vi "Device.Init.vi"(8 "error in (no error)":errorcluster, 11 "LIA.SR810":refnum<class "LIA.SR810.lvclass">) -> (0 "error out":errorcluster, 2 "Result":bool, 3 "LIA.SR810 out":refnum<class "LIA.SR810.lvclass">)   [LabVIEW 2017, in "LIA.SR810.lvclass"]
doc: "---------------------------------------------------------------\nJKI State Machine Objects™\nhttp://jki.net/state-machine-objects/\nCopyright (C) 2005-2015, JKI <info@jki.net>\nALL RIGHTS RESERVEDJKI State Machine Objects (SMO) 1.0.0.5\nJKI - JKI\nCopyright (c) 2016, JKI"
uses:
  LIA.SR810.lvclass
  D:/upwork/Laser Measurement Tool/Laser/project/Subsystems/LIA/LIA.lvclass
  Typedefs/Resource--Cluster.ctl
  LIA/LIA.lvclass
  <instrlib>/Stanford Research 830/Stanford Research 830.lvlib
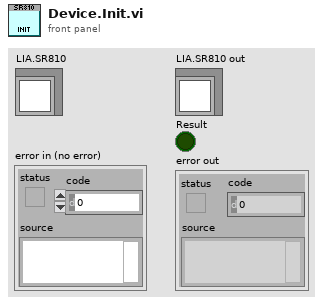
[diagram p1: front panel]
types:
  T1 = typedef "LIA.SR810.lvclass/Resource--Cluster.ctl" = cluster{"VISA resource":refnum<visa-resource-name>}
  T2 = typedef "LIA.lvclass/Configuration--Cluster.ctl" = cluster{"VISA Resource":string}
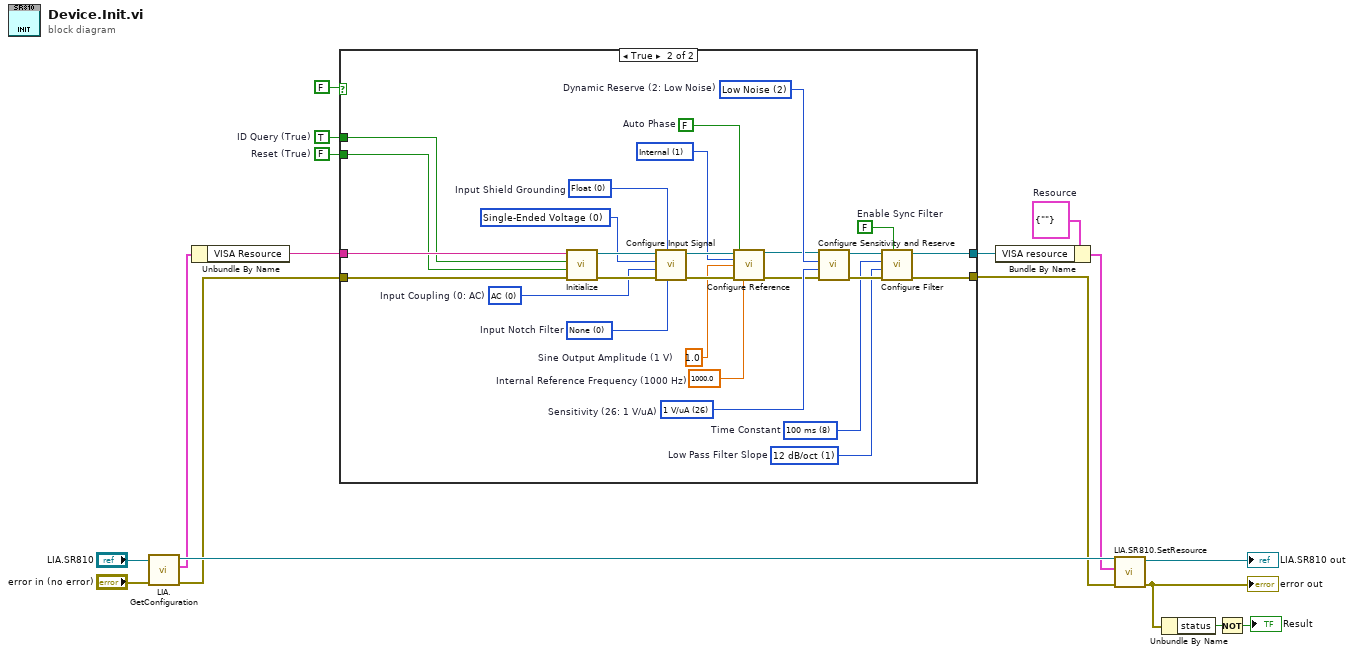
[diagram p0: block diagram]
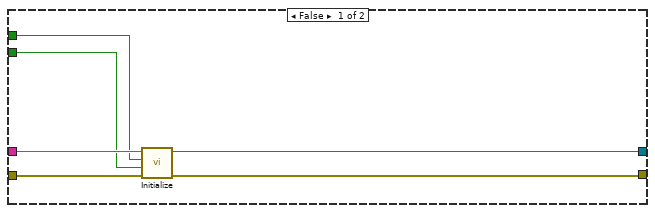
[diagram p2: hidden frame]
diagram:
  w5 = FALSE  # Reset (True)
  w6 = TRUE  # ID Query (True)
  w10 = T1 {"VISA resource"=""}  # Resource
  n1 = call "LIA.GetConfiguration.vi"("error in (no error)"="error in (no error)", "LIA"="LIA.SR810") -> ("error out"=w11:errorcluster, "Configuration"=w13:T2, "LIA out"=w14:refnum<class "LIA.SR810.lvclass">)  [unwired: 7 in]
  n2 = Unbundle By Name(w13) -> ("VISA Resource"=w12:string)
  n3 = case shown="True" FALSE {
    tunnel: w12 -> [w23 w29]
    tunnel: w11 -> [w22 w28]
    tunnel: [w20 w27] -> w9
    tunnel: [w21 w26] -> w8
    tunnel: w6 -> [w19 w25]
    tunnel: w5 -> [w18 w24]
    frame False {
      n4 = call <instrlib>:"Initialize.vi"("error in (no error)"=w22, "Reset (True)"=w18, "ID Query (True)"=w19, "VISA resource name"=w23) -> ("error out"=w21:errorcluster, "VISA resource name out"=w20:refnum<visa-resource-name>)  [unwired: 6 in]
    }
    frame True {
      w41 = i8 26 items=["Auto Gain"=-1, "2 nV/fA"=0, "5 nV/fA"=1, "10 nV/fA"=2, "20 nV/fA"=3, "50 nV/fA"=4, "100 nV/fA"=5, "200 nV/fA"=6, "500 nV/fA"=7, "1 uV/pA"=8, "2 uV/pA"=9, "5 uV/pA"=10, "10 uV/pA"=11, "20 uV/pA"=12, "50 uV/pA"=13, "100 uV/pA"=14, "200 uV/pA"=15, "500 uV/pA"=16, "1 mV/nA"=17, "2 mV/nA"=18, "5 mV/nA"=19, "10 mV/nA"=20, "20 mV/nA"=21, "50 mV/nA"=22, "100 mV/nA"=23, "200 mV/nA"=24, "500 mV/mA"=25, "1 V/uA"=26]  # Sensitivity (26: 1 V/uA)
      w35 = 1000.0  # Internal Reference Frequency (1000 Hz)
      w36 = 1.0  # Sine Output Amplitude (1 V)
      w45 = u16 0 items=["AC", "DC"]  # Input Coupling (0: AC)
      w46 = u16 0 items=["Single-Ended Voltage", "Differential Voltage", "1 MOhm Current Gain", "100 MOhm Current Gain"] ("Input Connection (0: Single-Ended Voltage)")
      w37 = u16 1 items=["External", "Internal"] ("Reference Source (1: Internal)")
      w40 = i8 2 items=["High Reserve"=0, "Normal"=1, "Low Noise"=2, "Auto Reserve"=-1]  # Dynamic Reserve (2: Low Noise)
      w30 = u16 1 items=["6 dB/oct", "12 dB/oct", "18 db/oct", "24 dB/oct"]  # Low Pass Filter Slope
      w31 = u16 8 items=["10 us", "30 us", "100 us", "300 us", "1 ms", "3 ms", "10 ms", "30 ms", "100 ms", "300 ms", "1 s", "3 s", "10 s", "30 s", "100 s", "300 s", "1 ks", "3 ks", "10 ks", "30 ks"]  # Time Constant
      w32 = FALSE  # Enable Sync Filter
      w42 = FALSE  # Auto Phase
      w43 = u16 0 items=["None", "Line Notch", "2x Line Notch", "Both Notch Filters"]  # Input Notch Filter
      w44 = u16 0 items=["Float", "Ground"]  # Input Shield Grounding
      n5 = call <instrlib>:"Initialize.vi"("error in (no error)"=w28, "Reset (True)"=w24, "ID Query (True)"=w25, "VISA resource name"=w29) -> ("error out"=w50:errorcluster, "VISA resource name out"=w49:refnum<visa-resource-name>)  [unwired: 6 in]
      n6 = call <instrlib>:"Configure Input Signal.vi"("Input Notch Filter (0: None)"=w43, "Input Shield Grounding (0: Float)"=w44, "error in (no error)"=w50, "Input Coupling (0: AC)"=w45, "Input Connection (0: Single-Ended Voltage)"=w46, "VISA resource name"=w49) -> ("error out"=w47:errorcluster, "VISA resource name out"=w48:refnum<visa-resource-name>)  [unwired: 4 in]
      n7 = call <instrlib>:"Configure Reference.vi"("VISA resource name"=w48, "Auto Phase (T: Enabled)"=w42, "Reference Source (1: Internal)"=w37, "Sine Output Amplitude (1 V)"=w36, "error in (no error)"=w47, "Internal Reference Frequency (1000 Hz)"=w35) -> ("VISA resource name out"=w39:refnum<visa-resource-name>, "error out"=w38:errorcluster)  [unwired: 8 in]
      n8 = call <instrlib>:"Configure Sensitivity and Reserve.vi"("error in (no error)"=w38, "Sensitivity (-1: Auto gain)"=w41, "Dynamic Reserve (-1: Auto Reserve)"=w40, "VISA resource name"=w39) -> ("error out"=w34:errorcluster, "VISA resource name out"=w33:refnum<visa-resource-name>)  [unwired: 6 in]
      n9 = call <instrlib>:"Configure Filter.vi"("Enable Sync Filter (F: Disable)"=w32, "error in (no error)"=w34, "Low Pass Filter Slope (1: 12dB/oct)"=w30, "Time Constant (8: 100ms)"=w31, "VISA resource name"=w33) -> ("error out"=w26:errorcluster, "VISA resource name out"=w27:refnum<visa-resource-name>)  [unwired: 5 in]
    }
  }
  n10 = Bundle By Name(cluster=w10, "VISA resource"=w9) -> (w7:T1)
  n11 = call "LIA.SR810.SetResource.vi"("error in (no error)"=w8, "Resource"=w7, "LIA.SR810 in"=w14) -> ("error out"=w2:errorcluster, "LIA.SR810 out"=→"LIA.SR810 out":refnum<class "LIA.SR810.lvclass">)  [unwired: 7 in]
  "error out" <- w2
  n12 = Unbundle By Name(w2) -> ("status"=w4:bool)
  n13 = Not(x=w4) -> (.not. x?=→"Result":bool)
